vi "Test cDAQ.vi"() -> ()   [LabVIEW 2020]
uses:
  Instruments/Pulse Driver/Pusle Driver Configuration.ctl
  <vilib>/DAQmx/create/channels.llb/DAQmx Create Channel (AI-Voltage-Basic).vi
  <vilib>/DAQmx/configure/timing.llb/DAQmx Timing (Sample Clock).vi
  <vilib>/DAQmx/configure/trigger.llb/DAQmx Reference Trigger (Digital Edge).vi
  <resource>/objmgr/daqmx.rc
  <vilib>/DAQmx/configure/events/hardwareSignals.llb/DAQmx Export Signal (Most Signals).vi
panel:
  in  "source":tag
  in  "error in":errorcluster
  in  "Samples per channel":i32=10000
  in  "Pretrigger samples":u32=1000
  out "task out":refnum<k21>
  in  "Pulse Configuration":T1={"Pre-trigger duration"=0.01, "Post-trigger duration"=0.1, "Rate"=1000000.0, "Ranges"=[10.0], "Re-name channels"=[], "Active channels"="0:1", "External clock"=FALSE} {"Rate" format="%#_8pHz"; "Post-trigger duration" format="%#_6ps"; "Pre-trigger duration" format="%#_6ps"; "Ranges" format="%#_6pV"}
  in  "DAQmx Device Name":tag="cDAQ1Mod1"
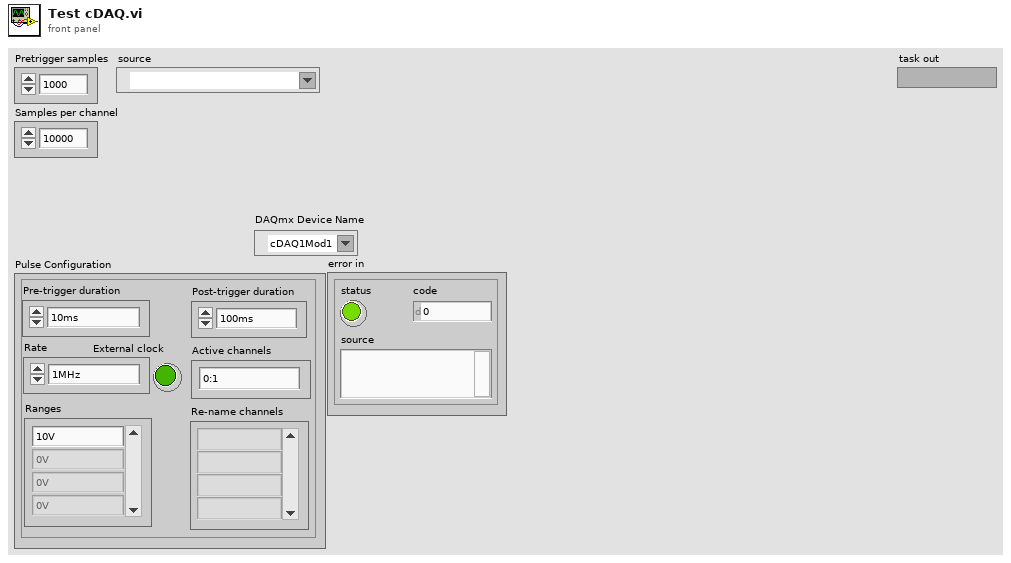
[diagram p1: front panel]
types:
  T1 = typedef "Pusle Driver Configuration.ctl" = cluster{"Pre-trigger duration":dbl, "Post-trigger duration":dbl, "Rate":dbl, "Ranges":dbl[], "Re-name channels":string[], "Active channels":string, "External clock":bool}
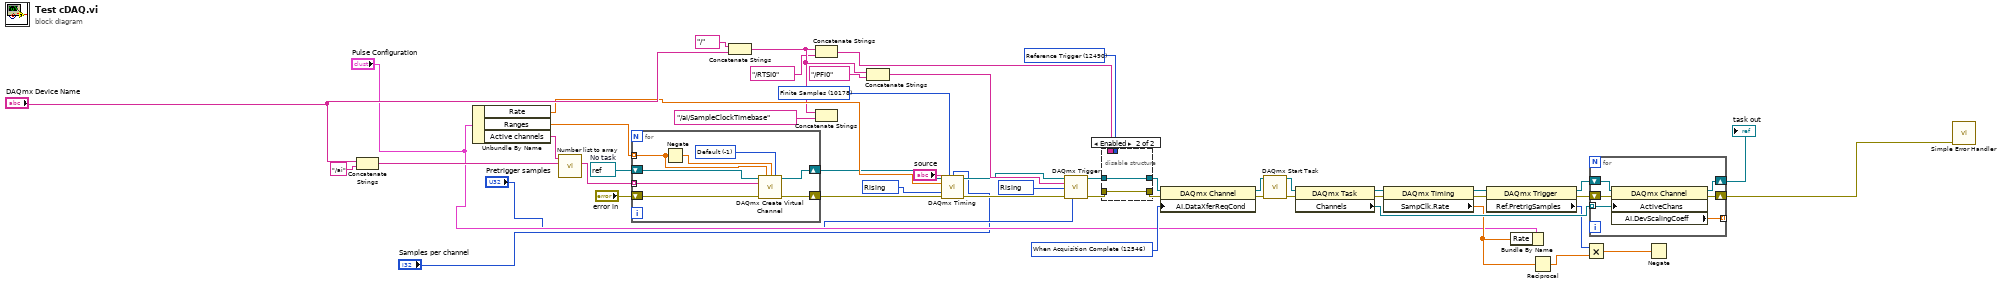
[diagram p0: block diagram]
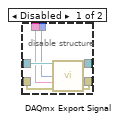
[diagram p2: hidden frame]
diagram:
  w6 = 12546 items=["Onboard Memory More than Half Full"=10237, "Onboard Memory Not Empty"=10241, "Onboard Memory Custom Threshold"=12577, "When Acquisition Complete"=12546] ("AI.DataXferReqCond")
  w17 = 12490 items=["AI Convert Clock"=12484, "10MHz Reference Clock"=12536, "20MHz Timebase Clock"=12486, "Sample Clock"=12487, "Advance Trigger"=12488, "Reference Trigger"=12490, "Start Trigger"=12491, "Advance Complete Event"=12492, "AI Hold Complete Event"=12493, "Counter Output Event"=12494, "Change Detection Event"=12511, "Watchdog Timer Expired Event"=12512] ("signal")
  w36 = refnum<k21> refnum  # No task
  w42 = 10280 items=["Rising"=10280, "Falling"=10171] ("active edge")
  w43 = 10178 items=["Finite Samples"=10178, "Continuous Samples"=10123, "Hardware Timed Single Point"=12522] ("sample mode")
  w49 = 10280 items=["Rising"=10280, "Falling"=10171] ("edge")
  n1 = Concatenate Strings("DAQmx Device Name", "/ai" ("string")) -> (w37:string)
  n2 = Unbundle By Name("Pulse Configuration") -> ("Rate"=w34:dbl, "Ranges"=w29:dbl[], "Active channels"=w39:string)
  n3 = call "Number list to array.vi"("Full names prefix"=w37, "Number list"=w39) -> ("Full names"=w35:string[])  [unwired: 8 in, 1 out]
  n4 = for {
    tunnel: w35 -> [w58] mode=indexing
    tunnel: w29 -> [w56] mode=indexing
    shift-right: [w53] -> w48
    shift-left: "error in" -> [w57]
    shift-right: [w54] -> w27
    shift-left: w36 -> [w51]
    w52 = -1 items=["Default"=-1, "RSE"=10083, "NRSE"=10078, "Differential"=10106, "Pseudodifferential"=12529] ("input terminal configuration")
    n5 = Negate(x=w56) -> (-x=w55:dbl)
    n6 = call-poly <vilib>:"DAQmx Create Virtual Channel.vi"("task in"=w51, "maximum value"=w56, "minimum value"=w55, "input terminal configuration"=w52, "physical channels"=w58, "error in"=w57) -> ("task out"=w54:refnum<k21>, "error out"=w53:errorcluster)  [unwired: 8 in]
  }
  n7 = Concatenate Strings(tag "/" ("string"), "DAQmx Device Name") -> (w11:string)
  n8 = Concatenate Strings(w11, tag "/RTSI0" ("string")) -> (w12:string)
  n9 = Concatenate Strings(w11, tag "/ai/SampleClockTimebase" ("string")) -> ()  [unwired: 1 out]
  n10 = Concatenate Strings(w11, tag "/PFI0" ("string")) -> (w47:string)
  n11 = call-poly <vilib>:"DAQmx Timing.vi"("task/channels in"=w27, "sample mode"=w43, "samples per channel"="Samples per channel", "rate"=w34, "source"="source", "active edge"=w42, "error in"=w48) -> ("task out"=w45:refnum<k21>, "error out"=w46:errorcluster)  [unwired: 7 out]
  n12 = call-poly <vilib>:"DAQmx Trigger.vi"("task/channels in"=w45, "source"=w47, "edge"=w49, "error in"=w46, "pretrigger samples per channel"="Pretrigger samples") -> ("task out"=w18:refnum<k21>, "error out"=w16:errorcluster)  [unwired: 9 out]
  n13 = disable-structure shown="Enabled" {
    disable-tunnel: w18 -> [w64 w65]
    disable-tunnel: w17 -> [w63 _]
    disable-tunnel: w16 -> [w62 w66]
    disable-tunnel: [w61 w66] -> w15
    disable-tunnel: w12 -> [w60 _]
    disable-tunnel: [w59 w65] -> w8
    frame Disabled {
      n14 = call-poly <vilib>:"DAQmx Export Signal.vi"("task/channels in"=w64, "signal"=w63, "output terminal"=w60, "error in"=w62) -> ("task out"=w59:refnum<k21>, "error out"=w61:errorcluster)  [unwired: 10 in]
    }
    frame Enabled {
    }
  }
  n15 = property class="DAQmx Channel"(reference=w8, error in=w15, "AI.DataXferReqCond"=w6) -> (reference out=w7:refnum<k21>, error out=w9:errorcluster)
  n16 = call <vilib>:"DAQmx Start Task.vi"("task/channels in"=w7, "error in"=w9) -> ("task out"=w41:refnum<k21>, "error out"=w40:errorcluster)  [unwired: 12 out]
  n17 = property class="DAQmx Task"(reference=w41, error in=w40) -> (reference out=w33:refnum<k21>, error out=w32:errorcluster, "Channels"=w28:refnum<k21>[])
  n18 = property class="DAQmx Timing"(reference=w33, error in=w32) -> (reference out=w25:refnum<k21>, error out=w22:errorcluster, "SampClk.Rate"=w26:dbl)
  n19 = property class="DAQmx Trigger"(reference=w25, error in=w22) -> (reference out=w24:refnum<k21>, error out=w23:errorcluster, "Ref.PretrigSamples"=w21:u32)
  n20 = Bundle By Name(cluster="Pulse Configuration", "Rate"=w26) -> ()  [unwired: 1 out]
  n21 = Reciprocal(x=w26) -> (1/x=w20:dbl)
  n22 = Multiply(x=w21, y=w20) -> (x*y=w19:dbl)
  n23 = for {
    tunnel: w28 -> [w72] mode=indexing
    shift-right: [w69] -> w31
    shift-left: w24 -> [w70]
    shift-right: [w68] -> w30
    shift-left: w23 -> [w71]
    tunnel: [w67] -> _ mode=indexing
    n24 = property class="DAQmx Channel"(reference=w70, error in=w71, "ActiveChans"=w72) -> (reference out=w69:refnum<k21>, error out=w68:errorcluster, "AI.DevScalingCoeff"=w67:dbl[])
  }
  "task out" <- w31
  n25 = Negate(x=w19) -> ()  [unwired: 1 out]
  n26 = call <vilib>:"Simple Error Handler.vi"("error in (no error)"=w30) -> ()  [unwired: 4 in, 5 out]
